vi "Model Index to String.vi"(10 "Code":u16 caption="代码") -> (2 "Info String":string caption="信息")   [LabVIEW 2023, in "Longer Pump dLSP501 Series.lvlib"]
uses:
  <instrlib>/Longer Pump dLSP501 Modbus RTU Series/Longer Pump dLSP501 Series.lvlib
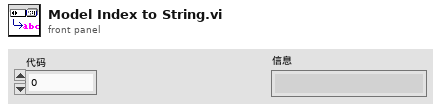
[diagram p1: front panel]
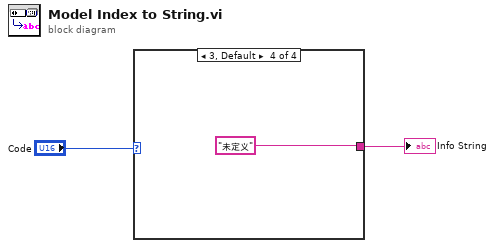
[diagram p0: block diagram]
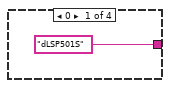
[diagram p2: hidden frame]
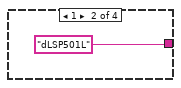
[diagram p3: hidden frame]
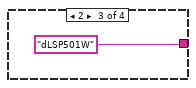
[diagram p4: hidden frame]
diagram:
  n1 = case shown="3, Default" "Code" {
    tunnel: ["dLSP501S" "dLSP501L" "dLSP501W" "未定义"] -> w2
    frame 0 {
    }
    frame 1 {
    }
    frame 2 {
    }
    frame 3, Default {
    }
  }
  "Info String" <- w2
